vi "CSTK_Enum_Creator_AttributeChanges.vi"(6 "标签名":string, 8 "错误输入（无错误）":errorcluster, 9 "项名":string, 10 "Enum输入":refnum<vi>, 11 "VI输入":refnum<vi>) -> (0 "错误输出":errorcluster, 2 "Enum输出":refnum<vi>, 3 "VI输出":refnum<vi>)   [LabVIEW 2015, in "CSTK_Enum Creator.lvlib"]
uses:
  CSTK_Enum Creator.lvlib
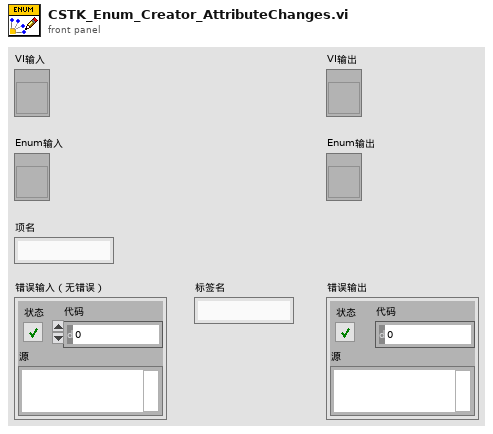
[diagram p1: front panel]
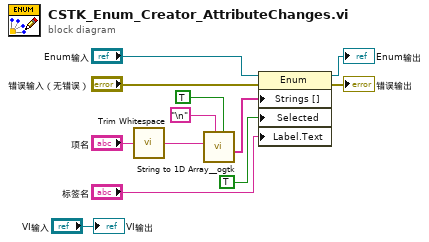
[diagram p0: block diagram]
diagram:
  n1 = call <vilib>:"Trim Whitespace.vi"("string"="项名") -> ("trimmed string"=w7:string)  [unwired: 1 in]
  n2 = call <userlib>:"String to 1D Array__ogtk.vi"("ignore duplicate delimiters? (F=No)"=TRUE, "delimiter (Tab)"="\n", "string"=w7) -> ("Array of Strings"=w10:string[])  [unwired: 8 in]
  n3 = property class="Enum"(reference="Enum输入", error in="错误输入（无错误）", "Strings []"=w10, "Selected"=TRUE ("选中"), "Label.Text"="标签名") -> (reference out=→"Enum输出":refnum<vi>, error out=→"错误输出":errorcluster)
  "VI输出" <- "VI输入"
